vi "API ID.vi"(11 "Event API in":refnum<class "EventAPI.lvclass">) -> (2 "ID":string)   [LabVIEW 2020, in "Volatus.lvlib" / "EventAPI.lvclass"]
uses:
  EventAPI.lvclass
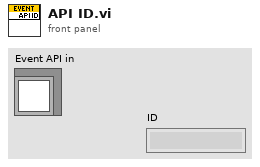
[diagram p1: front panel]
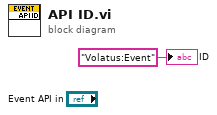
[diagram p0: block diagram]
diagram:
  "ID" <- "Volatus:Event" ("ID")
